vi "Destroy.vi"(11 "TEMPLATE jettl in":refnum<class "TEMPLATE jettl.lvclass">) -> (3 "TEMPLATE jettl out":refnum<class "TEMPLATE jettl.lvclass">)   [LabVIEW 2021, in "_Template.lvlib" / "Templates.lvlib" / "TEMPLATE jettl.lvlib" / "TEMPLATE jettl.lvclass"]
uses:
  TEMPLATE jettl.lvclass
  TEMPLATE jettl.lvclass/TEMPLATE jettl.ctl
  jettl/jettl/jettl/jettl.lvclass
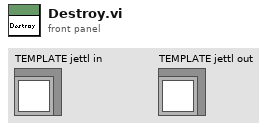
[diagram p1: front panel]
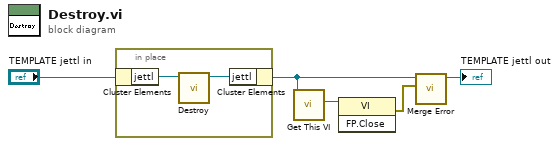
[diagram p0: block diagram]
diagram:
  n1 = in-place {
    n2 = in-place-cluster #1("TEMPLATE jettl in") -> ("jettl"=w7:refnum<class "jettl.lvclass">)
    n3 = call-dynamic "Destroy.vi"("jettl in"=w7) -> ("jettl out"=w6:refnum<class "jettl.lvclass">)  [unwired: 10 in]
    n4 = in-place-cluster #1("jettl"=w6) -> (w2:refnum<class "TEMPLATE jettl.lvclass">)
  }
  n5 = call-dynamic "Get This VI.vi"("TEMPLATE jettl in"=w2) -> ("This VI"=w4:refnum<vi>)  [unwired: 10 in]
  n6 = invoke class="VI" method="FP.Close"(reference=w4) -> (error out=w3:errorcluster)  [unwired: 2 in, 2 out]
  n7 = call-dynamic "Merge Error.vi"("Error"=w3, "TEMPLATE jettl in"=w2) -> ("TEMPLATE jettl out"=→"TEMPLATE jettl out":refnum<class "TEMPLATE jettl.lvclass">)  [unwired: 9 in]
